vi "AOL Control-4ch_common_CT.vi"() -> ()   [LabVIEW 2020]
uses:
  TypeDef/Frequency-4ch.ctl
  TypeDef/Amplitude-4ch.ctl
  Globals/FPGA Globals.vi
  <vilib>/DAQmx/create/channels.llb/DAQmx Create Channel (CO-Pulse Generation-Time).vi
  <vilib>/FPGAPlugInAG/PXIe-7976R/niLvFpga_Open_PXIe-7976R.vi
  <vilib>/rvi/interface/common/dynamic/niFpgaDynamicAddResources.vi
  <vilib>/FPGAPlugInAG/PXIe-7975R/niLvFpga_Open_PXIe-7975R.vi
  <vilib>/Utility/error.llb/Error Cluster From Error Code.vi
  <vilib>/rvi/errors/niLvFpgaAdjustHostInterfaceError.vi
  <vilib>/FPGAPlugInAG/Dynamic/niLvFpga_Close_Dynamic.vi
  <vilib>/rvi/interface/nirviOpenFPGA/nirviOpenFPGA.xnode
  FPGA Bitfiles/aolcontrolprojec_FPGATarget_Gentrigpulse_cQn7vg9KkEk.lvbitx
  FPGA Bitfiles/aolcontrolprojec_FPGATarget_Gentrigpulse_Cnv+VIMB-cw_AC.lvbitx
  FPGA Bitfiles/aolcontrolprojec_FPGATarget2_GenTrigPulse7975_JoXGkHjNmUo.lvbitx
  <vilib>/rvi/interface/nirviReadWriteControl/nirviReadWriteControl.xnode
  <vilib>/rvi/interface/nirviCloseFPGA/nirviCloseFPGA.xnode
  NiFpgaLv.dll
  <vilib>/rvi/interface/Simulation/niFpgaSimulationCallBeginRW.vi
panel:
  in  "Tab Control":T1(tab)
  in  "Use RF from file":bool
  in  "RF Code File":path=path "D:/Microscope data/2019-04-16/Sameer/Packets"
  in  "Frequency (MHz)":T2={"Ch 1"=39, "Ch 2"=39, "Ch 3"=39, "Ch 4"=39} {"Ch 4" min=20 max=50 step=1; "Ch 3" min=20 max=50 step=1; "Ch 2" min=20 max=50 step=1; "Ch 1" min=20 max=50 step=1}
  in  "Amplitude":T3={"Ch 1"=255, "Ch 2"=255, "Ch 3"=255, "Ch 4"=255} {"Ch 4" max=255 step=1; "Ch 3" max=255 step=1; "Ch 2" max=255 step=1; "Ch 1" max=255 step=1}
  in  "Stop":bool
  in  "Load":bool
  in  "Run":bool
  in  "Clear":bool
  in  "Settings":bool
  out "Ethernet Port Opened":bool
  out "RF Loaded":bool
  out "Trigger Sent":bool
  out "Status":string
  in  "Use detected RIO resource":bool
  in  "RIO Resource Name":string
  out "Detected RIO Resource Name":string
  in  "Use FlexRIO Trigger":bool=TRUE
  in  "DAQmx Trigger Channel":tag="PXI1Slot4/ctr0"
  in  "Pulse Width (sec)":dbl=1e-05
  in  "Initial Delay(sec)":dbl=0.01 format="%.6f"
  in  "FPGA Card":enum16{"7976R", "7975R"}(ring)
  in  "Adapter Module":enum16{"5772-DC", "5772-AC"}(ring)
  out "PC Mac Address":string caption="PC MAC Address"
  out "Select Device 1":i32=1 caption="Device 1 Port" min=1 max=5 step=1
  out "Select Device 2":i32=1 caption="Device 2 Port" min=1 max=5 step=1
  out "Packet Array":string[](array[string])
  out "No of Packets":i32
  out "FPGA MAC 1":string caption="Device 1 MAC Address"
  out "FPGA MAC 2":string caption="Device 2 MAC Address"
  out "Trigger Error":errorcluster
  in  "error in":errorcluster
  # "User needs to send a single TTL rising edge for the controller to generate RF."
  # "Trigger"
  # "Ethernet"
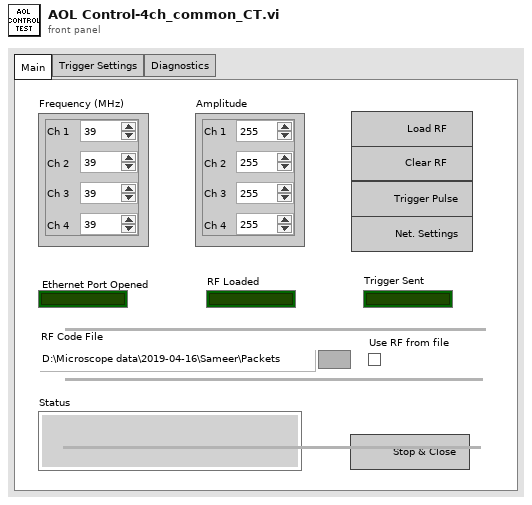
[diagram p1: front panel]
types:
  T1 = enum32{"Main", "Trigger Settings", "Diagnostics"}
  T2 = typedef "Frequency-4ch.ctl" = cluster{"Ch 1":u16, "Ch 2":u16, "Ch 3":u16, "Ch 4":u16}
  T3 = typedef "Amplitude-4ch.ctl" = cluster{"Ch 1":u16, "Ch 2":u16, "Ch 3":u16, "Ch 4":u16}
  T4 = enum8{"Enabled", "Disabled", "Disabled and Grayed Out"}
  T5 = typedef "FPGA Settings.ctl" = cluster{"System Clock(MHz)":dbl, "FPGA MAC 1":string, "Port Number 1":i32, "Port Number 2":i32, "FPGA MAC 2":string, "PC MAC Address":string}
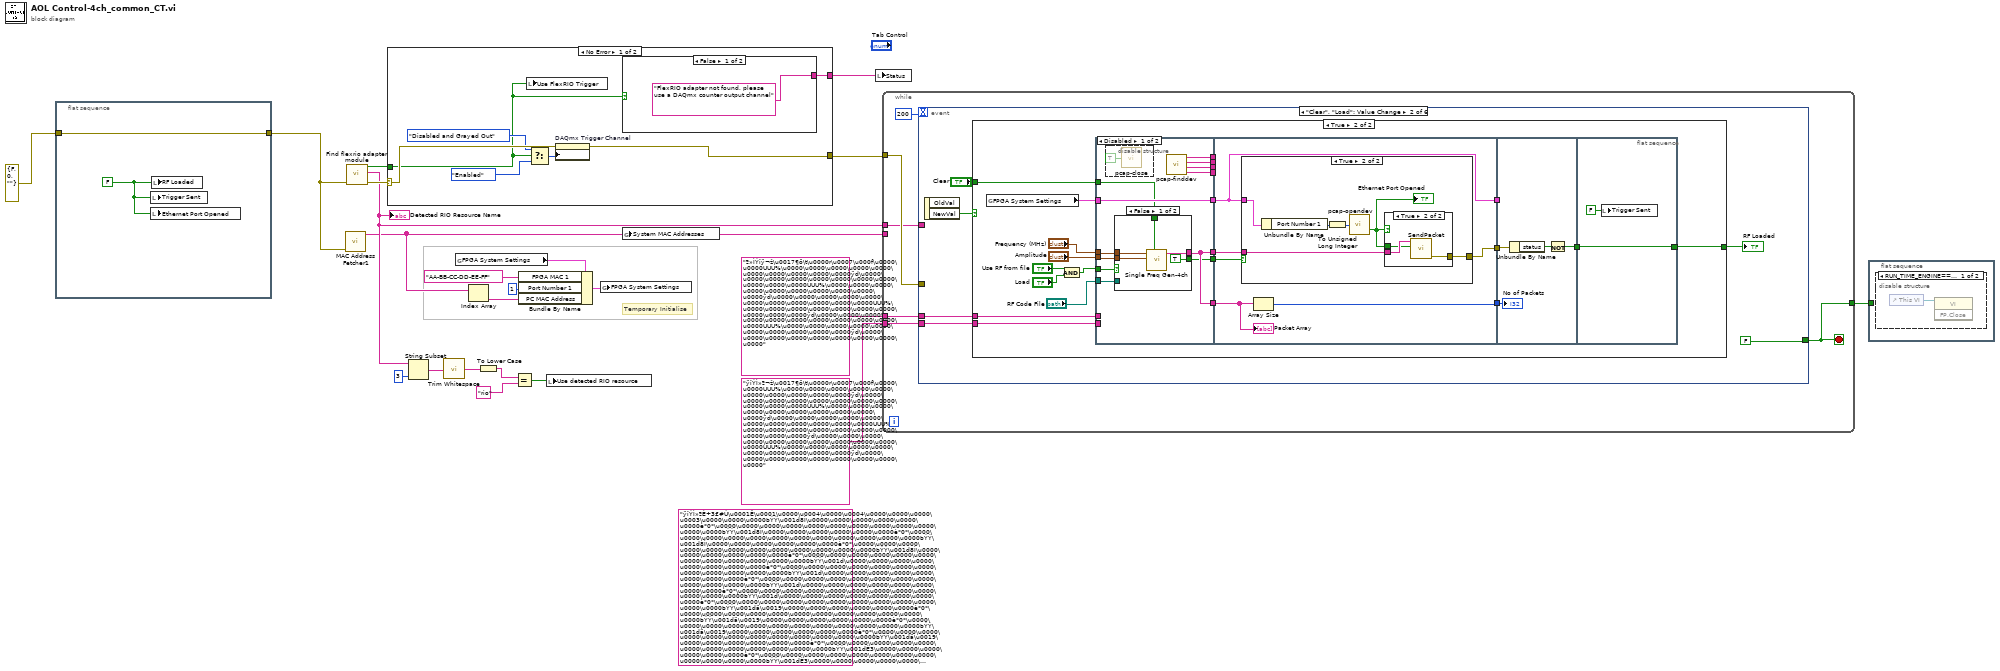
[diagram p0: block diagram]
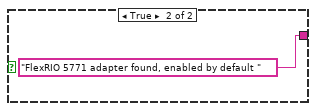
[diagram p2: hidden frame]
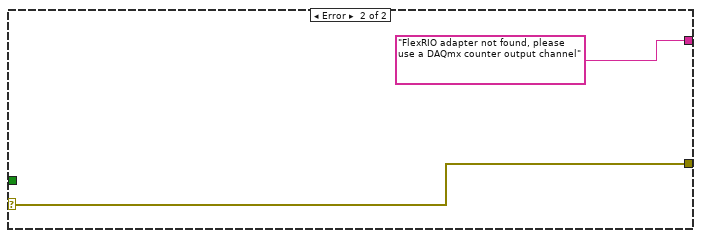
[diagram p3: hidden frame]
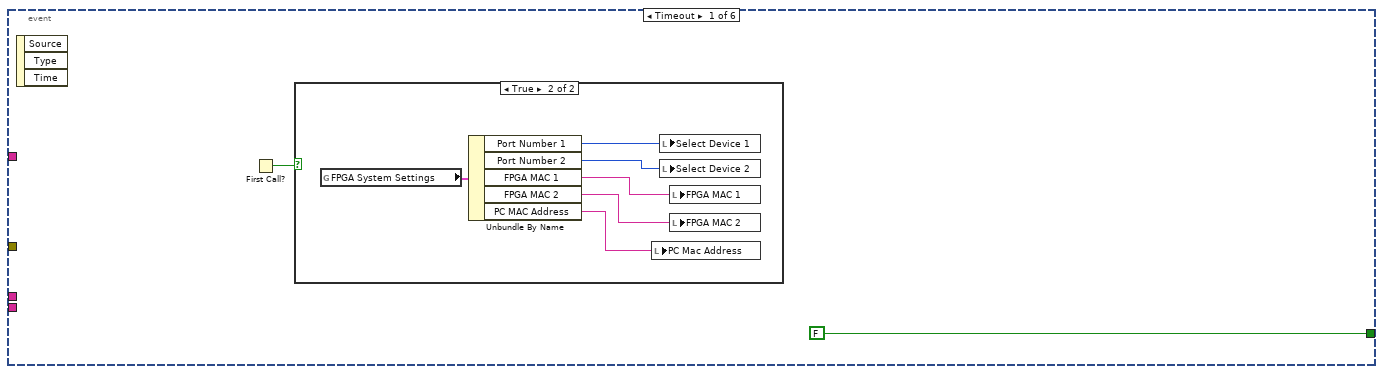
[diagram p5: hidden frame]
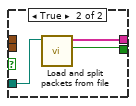
[diagram p8: hidden frame]
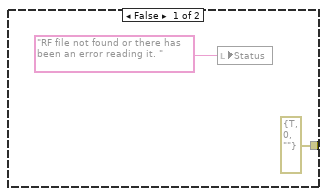
[diagram p10: hidden frame]
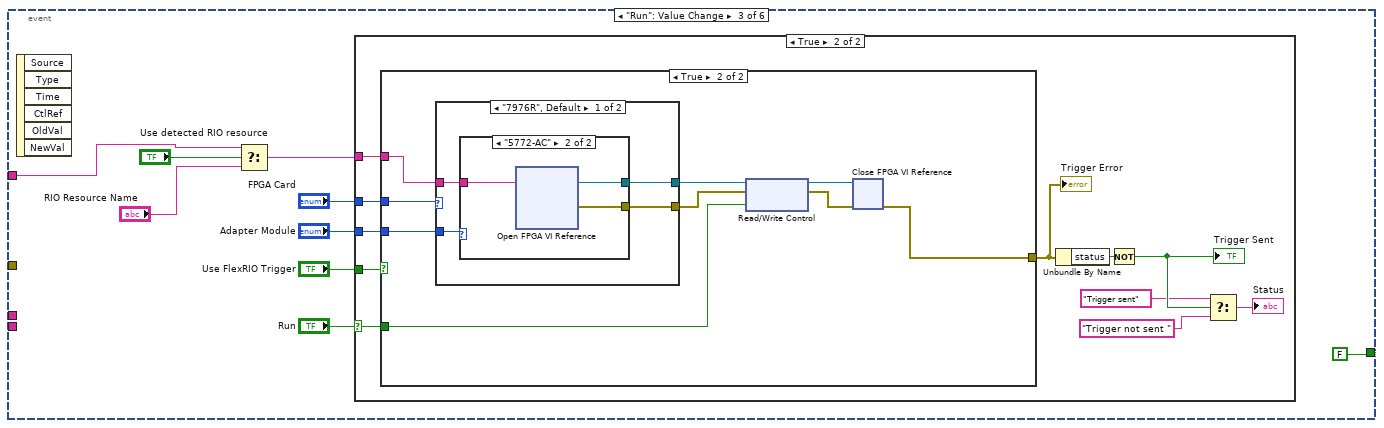
[diagram p12: hidden frame]
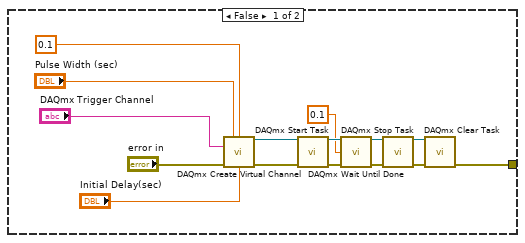
[diagram p14: hidden frame]
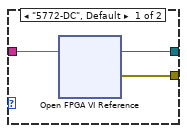
[diagram p15: hidden frame]
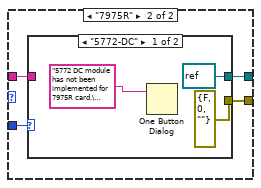
[diagram p16: hidden frame]
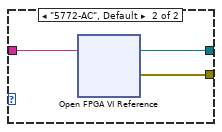
[diagram p17: hidden frame]
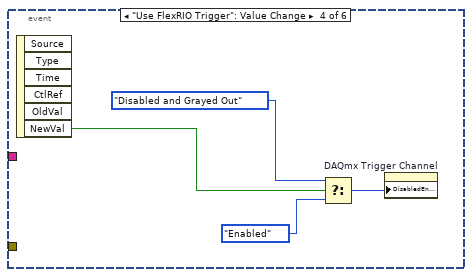
[diagram p18: hidden frame]
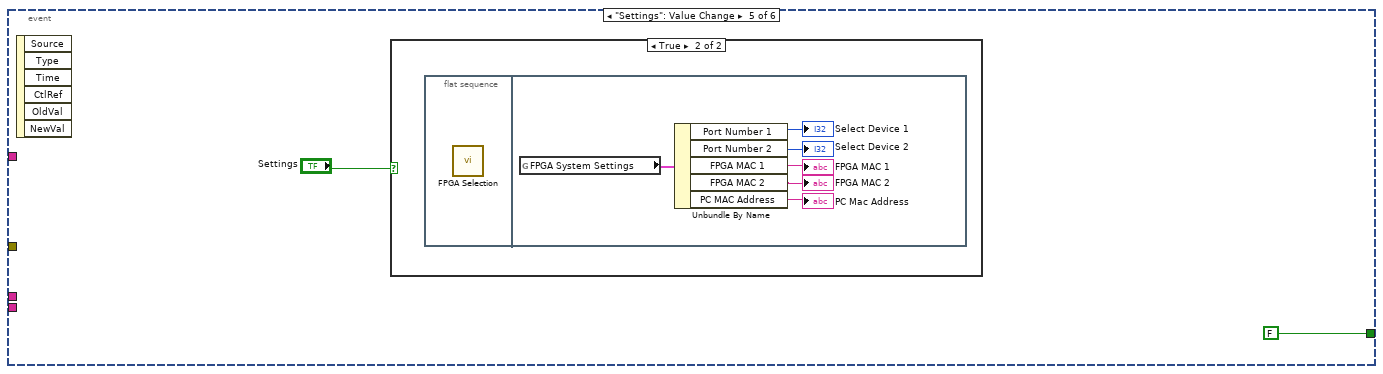
[diagram p19: hidden frame]
diagram:
  (unwired) "ÿîÝÌ»ªÈ÷3£#Ù\u0001Ê\u0001\u0000\u0004\u0000\u0004\u0000\u0000\u0000\u0003\u0000\u0000\u0000ÞÝÝ\u001d8Ì\u0000\u0000\u0000\u0000\u0000\u0000è*0*\u0000\u0000\u0000\u0000\u0000\u0000\u0000\u0000\u0000\u0000\u0000\u0000ÞÝÝ\u001d8Ì\u0000\u0000\u0000\u0000\u0000\u0000è*0*\u0000\u0000\u0000\u0000\u0000\u0000\u0000\u0000\u0000\u0000\u0000\u0000ÞÝÝ\u001d8Ì\u0000\u0000\u0000\u0000\u0000\u0000è*0*\u0000\u0000\u0000\u0000\u0000\u0000\u0000\u0000\u0000\u0000\u0000\u0000ÞÝÝ\u001d8Ì\u0000\u0000\u0000\u0000\u0000\u0000è*0*\u0000\u0000\u0000\u0000\u0000\u0000\u0000\u0000\u0000\u0000\u0000\u0000ÞÝÝ\u001d\u0000\u0000\u0000\u0000\u0000\u0000\u0000\u0000è*0*\u0000\u0000\u0000\u0000\u0000\u0000\u0000\u0000\u0000\u0000\u0000\u0000ÞÝÝ\u001d\u0000\u0000\u0000\u0000\u0000\u0000\u0000\u0000è*0*\u0000\u0000\u0000\u0000\u0000\u0000\u0000\u0000\u0000\u0000\u0000\u0000ÞÝÝ\u001d\u0000\u0000\u0000\u0000\u0000\u0000\u0000\u0000è*0*\u0000\u0000\u0000\u0000\u0000\u0000\u0000\u0000\u0000\u0000\u0000\u0000ÞÝÝ\u001d\u0000\u0000\u0000\u0000\u0000\u0000\u0000\u0000è*0*\u0000\u0000\u0000\u0000\u0000\u0000\u0000\u0000\u0000\u0000\u0000\u0000ÞÝÝ\u001dä\u0019\u0000\u0000\u0000\u0000\u0000\u0000è*0*\u0000\u0000\u0000\u0000\u0000\u0000\u0000\u0000\u0000\u0000\u0000\u0000ÞÝÝ\u001dä\u0019\u0000\u0000\u0000\u0000\u0000\u0000è*0*\u0000\u0000\u0000\u0000\u0000\u0000\u0000\u0000\u0000\u0000\u0000\u0000ÞÝÝ\u001dä\u0019\u0000\u0000\u0000\u0000\u0000\u0000è*0*\u0000\u0000\u0000\u0000\u0000\u0000\u0000\u0000\u0000\u0000\u0000\u0000ÞÝÝ\u001dä\u0019\u0000\u0000\u0000\u0000\u0000\u0000è*0*\u0000\u0000\u0000\u0000\u0000\u0000\u0000\u0000\u0000\u0000\u0000\u0000ÞÝÝ\u001dÈ3\u0000\u0000\u0000\u0000\u0000\u0000è*0*\u0000\u0000\u0000\u0000\u0000\u0000\u0000\u0000\u0000\u0000\u0000\u0000ÞÝÝ\u001dÈ3\u0000\u0000\u0000\u0000\u0000\u0000è*0*\u0000\u0000\u0000\u0000\u0000\u0000\u0000\u0000\u0000\u0000\u0000\u0000ÞÝÝ\u001dÈ3\u0000\u0000\u0000\u0000\u0000\u0000è*0*\u0000\u0000\u0000\u0000\u0000\u0000\u0000\u0000\u0000\u0000\u0000\u0000ÞÝÝ\u001dÈ3\u0000\u0000\u0000\u0000\u0000\u0000è*0*\u0000\u0000\u0000\u0000\u0000\u0000\u0000\u0000\u0000\u0000"
  # "Temporary Initialise"
  n1 = flat-sequence {
    tunnel: [w24] -> w14
    tunnel: errorcluster {"status"=FALSE, "code"=0, "source"=""} ("error in (no error)") -> [w24]
    frame #0 {
      w23 = FALSE ("RF Loaded")
      n2 = local write "Trigger Sent"(w23) -> ()
      n3 = local write "Ethernet Port Opened"(w23) -> ()
      n4 = local write "RF Loaded"(w23) -> ()
    }
  }
  n5 = call "MAC Address Fetcher1.vi"("error in (no error)"=w14) -> ("MAC Addresses"=w2:string[])  [unwired: 8 in, 2 out]
  n6 = call "Find flexrio adapter module.vi"("error in (no error)"=w14) -> ("error out"=w19:errorcluster, "Devices & Chassis:Provides Link Name"=w7:string, "NI 5772 adapter present ?"=w17:bool)  [unwired: 8 in]
  "Detected RIO Resource Name" <- w7
  n7 = case shown="No Error" w19 {
    selector: w19 -> [w31 w35]
    tunnel: w17 -> [w26 _]
    tunnel: [w27 w35] -> w18
    tunnel: [w25 "FlexRIO adapter not found, please use a DAQmx counter output channel"] -> w16
    frame No Error {
      n8 = local write "Use FlexRIO Trigger"(w26) -> ()
      n9 = Select(t=T4."Disabled and Grayed Out" ("Disabled"), s=w26, f=T4."Enabled") -> (s? t:f=w29:T4)
      n10 = property on="DAQmx Trigger Channel" class="DAQmxName"(error in=w31, "DisabledEnum"=w29) -> (error out=w27:errorcluster)  [unwired: 1 in, 1 out]
      n11 = case shown="False" w26 {
        tunnel: ["FlexRIO adapter not found, please use a DAQmx counter output channel" "FlexRIO 5771 adapter found, enabled by default "] -> w25
        frame False {
        }
        frame True {
        }
      }
    }
    frame Error {
    }
  }
  n12 = String Subset(string=w7, length (rest)=3 ("length (rest)")) -> (substring=w12:string)  [unwired: 1 in]
  n13 = call <vilib>:"Trim Whitespace.vi"("string"=w12) -> ("trimmed string"=w11:string)  [unwired: 1 in]
  n14 = global read "FPGA Globals.vi" "FPGA System Settings"() -> (w6:T5)
  n15 = Index Array(array=w2) -> (element=w1:string)  [unwired: 1 in]
  n16 = To Lower Case(string=w11) -> (all lower case string=w10:string)
  n17 = Equal?(x=w10, y="rio") -> (x = y?=w8:bool)
  n18 = Bundle By Name(cluster=w6, "FPGA MAC 1"="AA-BB-CC-DD-EE-FF" ("FPGA MAC 3"), "Port Number 1"=1, "PC MAC Address"=w1) -> (w3:T5)
  n19 = local write "Use detected RIO resource"(w8) -> ()
  n20 = global write "FPGA Globals.vi" "FPGA System Settings"(w3) -> ()
  n21 = global write "FPGA Globals.vi" "System MAC Addresses"(w2) -> ()
  n22 = local write "Status"(w16) -> ()
  n23 = while {
    tunnel: w2 -> [_]
    tunnel: "ª»ÌÝîÿ¬ž\u0017¶ö\t\u0000r\u0007\u000f\u0000\u0000UUU%\u0000\u0000\u0000\u0000\u0000\u0000\u0000\u0000\u0000\u0000ÿd\u0000\u0000\u0000\u0000\u0000\u0000\u0000\u0000\u0000\u0000\u0000UUU%\u0000\u0000\u0000\u0000\u0000\u0000\u0000\u0000\u0000\u0000ÿd\u0000\u0000\u0000\u0000\u0000\u0000\u0000\u0000\u0000\u0000\u0000UUU%\u0000\u0000\u0000\u0000\u0000\u0000\u0000\u0000\u0000\u0000ÿd\u0000\u0000\u0000\u0000\u0000\u0000\u0000\u0000\u0000\u0000\u0000UUU%\u0000\u0000\u0000\u0000\u0000\u0000\u0000\u0000\u0000\u0000ÿd\u0000\u0000\u0000\u0000\u0000\u0000\u0000\u0000\u0000" ("String") -> [w40]
    tunnel: "ÿîÝÌ»ª¬ž\u0017¶ö\t\u0000r\u0007\u000f\u0000\u0000UUU%\u0000\u0000\u0000\u0000\u0000\u0000\u0000\u0000\u0000\u0000ÿd\u0000\u0000\u0000\u0000\u0000\u0000\u0000\u0000\u0000\u0000\u0000UUU%\u0000\u0000\u0000\u0000\u0000\u0000\u0000\u0000\u0000\u0000ÿd\u0000\u0000\u0000\u0000\u0000\u0000\u0000\u0000\u0000\u0000\u0000UUU%\u0000\u0000\u0000\u0000\u0000\u0000\u0000\u0000\u0000\u0000ÿd\u0000\u0000\u0000\u0000\u0000\u0000\u0000\u0000\u0000\u0000\u0000UUU%\u0000\u0000\u0000\u0000\u0000\u0000\u0000\u0000\u0000\u0000ÿd\u0000\u0000\u0000\u0000\u0000\u0000\u0000\u0000\u0000" ("String") -> [w39]
    tunnel: [w38] -> w20
    tunnel: w18 -> [w37]
    tunnel: w7 -> [w36]
    stop <- w38 stop-if-true
    n24 = event shown="[1] \"Clear\", \"Load\": Value Change" {
      selector: _ -> [_ _ _ _ _ _]
      dyn-events: _ -> [_ _ _ _ _ _]
      timeout: 200 -> [_ _ _ _ _ _]
      tunnel: w40 -> [_ w53 _ _ _ _]
      tunnel: w39 -> [_ w52 _ _ _ _]
      tunnel: [FALSE FALSE FALSE _ FALSE w199] -> w38
      tunnel: w37 -> [_ _ _ _ _ _]
      tunnel: w36 -> [_ _ w125 _ _ _]
      event Timeout {
        n25 = event-data() -> ()  [unwired: 1 in, 3 out]
        n26 = First Call?() -> (First Call?: T/F=w42:bool)
        n27 = case shown="True" w42 {
          frame False {
          }
          frame True {
            n28 = global read "FPGA Globals.vi" "FPGA System Settings"() -> (w49:T5)
            n29 = Unbundle By Name(w49) -> ("Port Number 1"=w48:i32, "Port Number 2"=w47:i32, "FPGA MAC 1"=w46:string, "FPGA MAC 2"=w45:string, "PC MAC Address"=w44:string)
            n30 = local write "PC Mac Address"(w44) -> ()
            n31 = local write "Select Device 1"(w48) -> ()
            n32 = local write "Select Device 2"(w47) -> ()
            n33 = local write "FPGA MAC 1"(w46) -> ()
            n34 = local write "FPGA MAC 2"(w45) -> ()
          }
        }
      }
      event "Clear", "Load": Value Change {
        n35 = event-data() -> ("NewVal"=w55:bool)  [unwired: 1 in, 1 out]
        n36 = case shown="True" w55 {
          tunnel: "Clear" -> [_ w71]
          tunnel: w53 -> [_ w66]
          tunnel: w52 -> [_ w65]
          tunnel: [_ w63] -> w50
          frame False {
          }
          frame True {
            n37 = global read "FPGA Globals.vi" "FPGA System Settings"() -> (w72:T5)
            n38 = And(x="Use RF from file", y="Load") -> (x .and. y?=w56:bool)
            n39 = flat-sequence {
              tunnel: "Amplitude" -> [w90]
              tunnel: "Frequency (MHz)" -> [w89]
              tunnel: [w88] -> w78
              tunnel: w72 -> [w88]
              tunnel: w71 -> [w87]
              tunnel: [w86] -> w70
              tunnel: [w85] -> w69
              tunnel: [w84] -> w68
              tunnel: [w83] -> w67
              tunnel: w66 -> [_]
              tunnel: w65 -> [_]
              tunnel: [w82] -> w64
              tunnel: [w82] -> w61
              tunnel: w56 -> [w81]
              tunnel: "RF Code File" -> [w80]
              tunnel: [w79] -> w59
              tunnel: [w105] -> w77
              tunnel: [w104] -> w76
              tunnel: w78 -> [w103]
              tunnel: [w103] -> w75
              tunnel: w70 -> [_]
              tunnel: w69 -> [_]
              tunnel: w68 -> [_]
              tunnel: w67 -> [_]
              tunnel: w64 -> [w102]
              tunnel: w61 -> [w101]
              tunnel: w59 -> [w100]
              tunnel: w77 -> [w119]
              tunnel: w76 -> [w120]
              tunnel: w75 -> [_]
              tunnel: [w117] -> w62
              tunnel: [w122] -> w63
              tunnel: w62 -> [w122]
              frame #0 {
                n40 = disable-structure shown="Disabled" {
                  frame Disabled {
                    n41 = call "pcap-close.vi"("Opened"=TRUE) -> ()
                  }
                  frame Enabled {
                  }
                }
                n42 = case shown="False" w81 {
                  tunnel: w90 -> [w95 _]
                  tunnel: w89 -> [w94 _]
                  tunnel: w87 -> [w93 _]
                  tunnel: [w92 w96] -> w82
                  tunnel: w80 -> [_ w98]
                  tunnel: [TRUE ("OK?") w97] -> w79
                  frame False {
                    n43 = call "Single Freq Gen-4ch.vi"("Stop Single Frquency"=w93, "Amplitude"=w95, "Frequency (MHz)"=w94) -> ("Hex String (Array)"=w92:string[])  [unwired: 7 in, 1 out]
                  }
                  frame True {
                    n44 = call "Load and split packets from file.vi"("Path"=w98) -> ("OK?"=w97:bool, "Hex String"=w96:string[])  [unwired: 7 in, 2 out]
                  }
                }
                n45 = call "pcap-finddev.vi"() -> ("String 4"=w83:string, "String 3"=w84:string, "String 2"=w85:string, "String"=w86:string)  [unwired: 1 in, 1 out]
              }
              frame #1 {
                n46 = case shown="True" w100 {
                  tunnel: [errorcluster {"status"=TRUE, "code"=0, "source"=""} ("error out") w113] -> w105
                  tunnel: w103 -> [_ w110]
                  tunnel: w102 -> [_ w108]
                  frame False {
                    n47 = local write "Status"("RF file not found or there has been an error reading it. " ("Status")) -> ()
                  }
                  frame True {
                    n48 = Unbundle By Name(w110) -> ("Port Number 1"=w112:i32)
                    n49 = To Unsigned Long Integer(number=w112) -> (unsigned 32bit integer=w111:u32)
                    n50 = call "pcap-opendev.vi"("Select Device"=w111) -> ("Opened"=w109:bool)  [unwired: 2 out]
                    "Ethernet Port Opened" <- w109
                    n51 = case shown="True" w109 {
                      tunnel: [_ w116] -> w113
                      tunnel: w108 -> [_ w115]
                      tunnel: w109 -> [_ w114]
                      frame False {
                      }
                      frame True {
                        n52 = call "SendPacket.vi"("Ethernet Port Opened ?"=w114, "Packet Array"=w115) -> ("error out"=w116:errorcluster)  [unwired: 8 in, 1 out]
                      }
                    }
                  }
                }
                n53 = Array Size(array=w101) -> (size(s)=w104:i32)
                "Packet Array" <- w101
              }
              frame #2 {
                n54 = Unbundle By Name(w119) -> ("status"=w118:bool)
                n55 = Not(x=w118) -> (.not. x?=w117:bool)
                "No of Packets" <- w120
              }
              frame #3 {
                n56 = local write "Trigger Sent"(FALSE ("Trigger Sent")) -> ()
              }
            }
          }
        }
        "RF Loaded" <- w50
      }
      event "Run": Value Change {
        n57 = event-data() -> ()  [unwired: 1 in, 6 out]
        n58 = Select(t=w125, s="Use detected RIO resource", f="RIO Resource Name") -> (s? t:f=w123:string)
        n59 = case shown="True" "Run" {
          selector: "Run" -> [_ w135]
          tunnel: "Use FlexRIO Trigger" -> [_ w142]
          tunnel: "FPGA Card" -> [_ w134]
          tunnel: "Adapter Module" -> [_ w133]
          tunnel: w123 -> [_ w132]
          frame False {
          }
          frame True {
            n60 = case shown="True" w142 {
              tunnel: [w143 w161] -> w141
              tunnel: w135 -> [_ w164]
              tunnel: w134 -> [_ w160]
              tunnel: w133 -> [_ w159]
              tunnel: w132 -> [_ w158]
              frame False {
                n61 = call-poly <vilib>:"DAQmx Create Virtual Channel.vi"("high time"="Pulse Width (sec)", "low time"=0.1 ("Pulse Low Time(sec)"), "counter"="DAQmx Trigger Channel", "error in"="error in", "initial delay"="Initial Delay(sec)") -> ("task out"=w152:refnum<k21>, "error out"=w151:errorcluster)  [unwired: 9 in]
                n62 = call <vilib>:"DAQmx Start Task.vi"("task/channels in"=w152, "error in"=w151) -> ("task out"=w150:refnum<k21>, "error out"=w146:errorcluster)  [unwired: 12 in]
                n63 = call <vilib>:"DAQmx Wait Until Done.vi"("task/channels in"=w150, "timeout (sec)"=0.1, "error in"=w146) -> ("task out"=w145:refnum<k21>, "error out"=w144:errorcluster)  [unwired: 11 in]
                n64 = call <vilib>:"DAQmx Stop Task.vi"("task/channels in"=w145, "error in"=w144) -> ("task out"=w149:refnum<k21>, "error out"=w148:errorcluster)  [unwired: 12 in]
                n65 = call <vilib>:"DAQmx Clear Task.vi"("task in"=w149, "error in"=w148) -> ("error out"=w143:errorcluster)  [unwired: 13 in]
              }
              frame True {
                n66 = case shown="\"7976R\", Default" w160 {
                  tunnel: [w170 w179] -> w166
                  tunnel: [w169 w178] -> w165
                  tunnel: w159 -> [w168 w180]
                  tunnel: w158 -> [w167 w177]
                  frame "7976R", Default {
                    n67 = case shown="\"5772-AC\"" w168 {
                      tunnel: [w173 w176] -> w170
                      tunnel: [w172 w175] -> w169
                      tunnel: w167 -> [w171 w174]
                      frame "5772-DC", Default {
                        n68 = xnode "Open FPGA VI Reference"("resource name"=w171) -> ("FPGA VI Reference Out"=w173:refnum<k20>, "error out"=w172:errorcluster)  [unwired: 1 in]
                      }
                      frame "5772-AC" {
                        n69 = xnode "Open FPGA VI Reference"("resource name"=w174) -> ("FPGA VI Reference Out"=w176:refnum<k20>, "error out"=w175:errorcluster)  [unwired: 1 in]
                      }
                    }
                  }
                  frame "7975R" {
                    n70 = case shown="\"5772-DC\"" w180 {
                      tunnel: [refnum<k20> refnum ("FPGA VI Reference Out") w186] -> w179
                      tunnel: [errorcluster {"status"=FALSE, "code"=0, "source"=""} ("error out") w185] -> w178
                      tunnel: w177 -> [_ w184]
                      frame "5772-DC" {
                        n71 = One Button Dialog(message="5772 DC module has not been implemented for 7975R card.\nPlease check your installed hardware. ") -> ()  [unwired: 1 in, 1 out]
                      }
                      frame "5772-AC", Default {
                        n72 = xnode "Open FPGA VI Reference"("resource name"=w184) -> ("FPGA VI Reference Out"=w186:refnum<k20>, "error out"=w185:errorcluster)  [unwired: 1 in]
                      }
                    }
                  }
                }
                n73 = xnode "Read/Write Control"("FPGA VI Reference In"=w166, "error in"=w165, "TL Input"=w164) -> ("FPGA VI Reference Out"=w163:refnum<k20>, "error out"=w162:errorcluster)
                n74 = xnode "Close FPGA VI Reference"("FPGA VI Reference In"=w163, "error in"=w162) -> ("error out"=w161:errorcluster)
              }
            }
            "Trigger Error" <- w141
            n75 = Unbundle By Name(w141) -> ("status"=w140:bool)
            n76 = Not(x=w140) -> (.not. x?=w139:bool)
            "Trigger Sent" <- w139
            n77 = Select(t="Trigger sent", s=w139, f="Trigger not sent ") -> (s? t:f=→"Status":string)
          }
        }
      }
      event "Use FlexRIO Trigger": Value Change {
        n78 = event-data() -> ("NewVal"=w190:bool)  [unwired: 1 in, 5 out]
        n79 = Select(t=T4."Disabled and Grayed Out" ("Disabled"), s=w190, f=T4."Enabled" ("Disabled")) -> (s? t:f=w187:T4)
        n80 = property on="DAQmx Trigger Channel" class="DAQmxName"("DisabledEnum"=w187) -> ()  [unwired: 2 in, 2 out]
      }
      event "Settings": Value Change {
        n81 = event-data() -> ()  [unwired: 1 in, 6 out]
        n82 = case shown="True" "Settings" {
          frame False {
          }
          frame True {
            n83 = flat-sequence {
              frame #0 {
                n84 = call "FPGA Selection.vi"() -> ()  [unwired: 12 in]
              }
              frame #1 {
                n85 = global read "FPGA Globals.vi" "FPGA System Settings"() -> (w196:T5)
                n86 = Unbundle By Name(w196) -> ("Port Number 1"=→"Select Device 1":i32, "Port Number 2"=→"Select Device 2":i32, "FPGA MAC 1"=→"FPGA MAC 1":string, "FPGA MAC 2"=→"FPGA MAC 2":string, "PC MAC Address"=→"PC Mac Address":string)
              }
            }
          }
        }
      }
      event "Stop": Value Change {
        n87 = event-data() -> ()  [unwired: 1 in, 6 out]
        n88 = local read "Ethernet Port Opened"() -> (w200:bool)
        n89 = flat-sequence {
          tunnel: w200 -> [w202]
          tunnel: [TRUE] -> w199
          frame #0 {
            n90 = call "pcap-close.vi"("Opened"=w202) -> ()
          }
        }
      }
    }
  }
  n91 = flat-sequence {
    tunnel: w20 -> [_]
    frame #0 {
      n92 = disable-structure shown="RUN_TIME_ENGINE==True" {
        frame condition #0 {
          n93 = control-ref of="This VI"() -> (w203:refnum<vi>)
          n94 = invoke class="VI" method="FP.Close"(reference=w203) -> ()  [unwired: 2 in, 3 out]
        }
        frame condition #1 (active) {
        }
      }
    }
  }
